vi "Generate Waveforms.vi"(5 "Number of Channels":i32, 6 "Frequencies":dbl[](array[numeric]), 7 "Sample Rate Hz":dbl, 8 "error in (no error)":errorcluster, 9 "Amplitudes":dbl[](array[numeric]), 10 "Samples Per Channel":i32, 11 "Total Samples":i64) -> (0 "error out":errorcluster, 2 "Total_Samples":i64, 3 "Waveforms":waveform(dbl)[](array[waveform]))   [LabVIEW 2026, in "Acquisition.lvlib"]
uses:
  Acquisition.lvlib
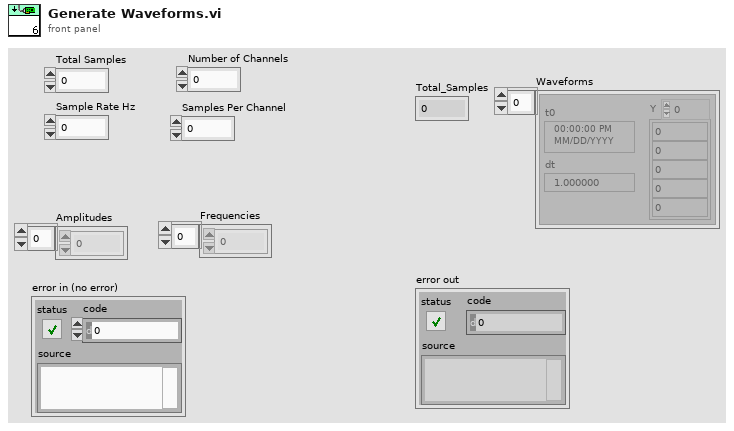
[diagram p1: front panel]
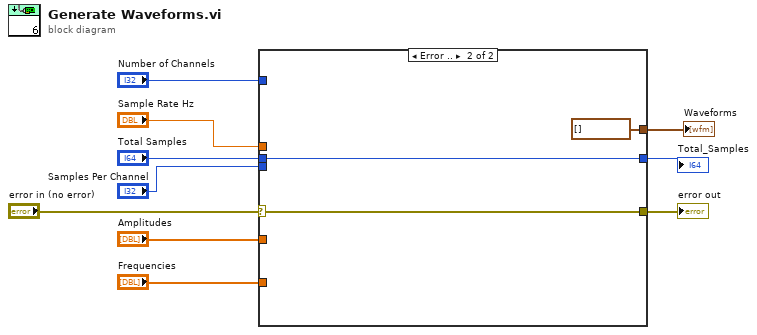
[diagram p0: block diagram]
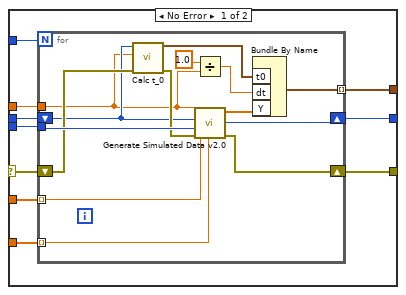
[diagram p2: hidden frame]
diagram:
  n1 = case shown="Error .." "error in (no error)" {
    selector: "error in (no error)" -> [w11 w37]
    tunnel: "Frequencies" -> [w20 _]
    tunnel: "Amplitudes" -> [w19 _]
    tunnel: "Number of Channels" -> [w18 _]
    tunnel: [w17 waveform(dbl)[] []] -> w7
    tunnel: [w16 w36] -> w6
    tunnel: "Samples Per Channel" -> [w15 _]
    tunnel: [w14 w37] -> w4
    tunnel: "Total Samples" -> [w13 w36]
    tunnel: "Sample Rate Hz" -> [w12 _]
    frame No Error {
      n2 = for {
        N: w18 -> [_]
        tunnel: w15 -> [w34]
        tunnel: w12 -> [w24]
        shift-right: [w26] -> w14
        shift-left: w11 -> [w28]
        shift-right: [w33] -> w16
        shift-left: w13 -> [w25]
        tunnel: [w30] -> w17 mode=indexing
        tunnel: w19 -> [w21] mode=indexing
        tunnel: w20 -> [w29] mode=indexing
        n3 = call "Calc t_0.vi"("error in (no error)"=w28, "Sample_Rate_Hz"=w24, "Total_Samples"=w25) -> ("error out"=w27:errorcluster, "t_0"=w22:timestamp)  [unwired: 7 in]
        n4 = Divide(x=1.0, y=w24) -> (x/y=w23:dbl)
        n5 = call "Generate Simulated Data v2.0.vi"("Frequency"=w29, "Amplitude"=w21, "error in (no error)"=w27, "Samples"=w34, "Total_Samples in"=w25, "Sample_Rate"=w24) -> ("error out"=w26:errorcluster, "Total_Samples out"=w33:i64, "Y"=w31:dbl[])  [unwired: 3 in]
        n6 = Bundle By Name("t0"=w22, "dt"=w23, "Y"=w31) -> (w30:waveform(dbl))  [unwired: 1 in]
      }
    }
    frame Error {
    }
  }
  "Waveforms" <- w7
  "Total_Samples" <- w6
  "error out" <- w4
